vi "calculate potential field.vi"(5 "vehicle Fx":fxp<+/-,16,13> format="%.7g", 7 "vehicle Fy":fxp<+/-,16,13> format="%.7g", 8 "F constant":i16, 9 "Is object?":bool, 10 "object distance squared":i16, 11 "angle":u8) -> (0 "F angle":i8, 1 "F magnitude":i16, 3 "scan complete?":bool)   [LabVIEW 2010]
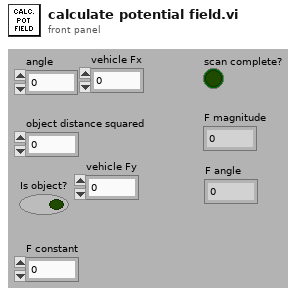
[diagram p1: front panel]
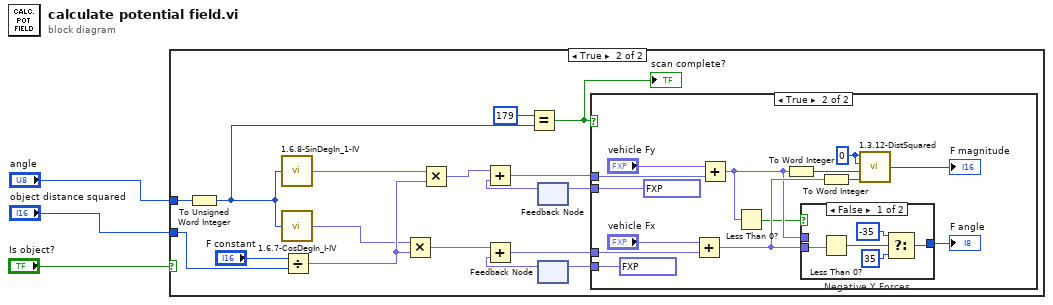
[diagram p0: block diagram]
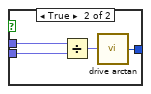
[diagram p4: hidden frame]
diagram:
  n1 = case shown="True" "Is object?" {
    tunnel: "angle" -> [_ w9]
    tunnel: "object distance squared" -> [_ w10]
    frame False {
    }
    frame True {
      n2 = To Unsigned Word Integer(number=w9) -> (unsigned 16bit integer=w6:u16)
      n3 = call "1.6.8-SinDegIn_1-IV.vi"("theta"=w6) -> ("Numeric"=w7:fxp<+/-,16,1>)
      n4 = call "1.6.7-CosDegIn_I-IV.vi"("theta"=w6) -> ("Numeric"=w8:fxp<+/-,16,1>)
      n5 = Divide(x="F constant", y=w10) -> (x/y=w12:fxp<+/-,32,16>)
      n6 = Multiply(x=w8, y=w12) -> (x*y=w13:fxp<+/-,48,17>)
      n7 = Multiply(x=w7, y=w12) -> (x*y=w14:fxp<+/-,48,17>)
      n8 = Equal?(x=u16 179, y=w6) -> (x = y?=w5:bool)
      "scan complete?" <- w5
      n9 = feedback #1() -> (w20:fxp<+/-,16,13>)  [unwired: 1 in]
      n10 = Add(x=w14, y=w20) -> (x+y=w18:fxp<+/-,16,13>)
      n11 = feedback #2() -> (w19:fxp<+/-,16,13>)  [unwired: 1 in]
      n12 = Add(x=w13, y=w19) -> (x+y=w17:fxp<+/-,16,13>)
      n13 = case shown="True" w5 {
        tunnel: w18 -> [w21 w29]
        tunnel: w17 -> [w22 w34]
        tunnel: [w22 fxp<+/-,16,13> 0.0] -> w16
        tunnel: [w21 fxp<+/-,16,13> 0.0] -> w15
        frame False {
        }
        frame True {
          w26 = i16 0 ("y position")
          n14 = Add(x="vehicle Fx", y=w34) -> (x+y=w31:fxp<+/-,17,14>)
          n15 = Add(x="vehicle Fy", y=w29) -> (x+y=w27:fxp<+/-,17,14>)
          n16 = Less Than 0?(x=w27) -> (x < 0?=w23:bool)
          n17 = To Word Integer(number=w27) -> (16bit integer=w24:i16)
          n18 = case "Negative Y Forces" shown="False" w23 {
            tunnel: [w37 w45] -> w32
            tunnel: w31 -> [w38 w44]
            tunnel: w27 -> [_ w43]
            frame False {
              n19 = Less Than 0?(x=w38) -> (x < 0?=w39:bool)
              n20 = Select(t=i8 -35 ("F angle"), s=w39, f=i8 35 ("F angle")) -> (s? t:f=w37:i8)
            }
            frame True {
              n21 = Divide(x=w43, y=w44) -> (x/y=w42:fxp<+/-,32,16>)
              n22 = call "drive arctan.vi"("x/y (tan)"=w42) -> ("Numeric 2"=w45:i8)
            }
          }
          "F angle" <- w32
          n23 = To Word Integer(number=w31) -> (16bit integer=w25:i16)
          n24 = call "1.3.12-DistSquared.vi"("x LIDAR position"=w25, "y LIDAR position"=w24, "x position"=w26, "y position"=w26) -> ("distance squared"=→"F magnitude":i16)  [unwired: 2 in]
        }
      }
      n25 = feedback-in #1(w15) -> ()
      n26 = feedback-in #2(w16) -> ()
    }
  }
